vi "MPUAutoReadOn.vi"(8 "ErrorIn(no error)":errorcluster, 10 "SampleRate(1000Hz)":u32=1000, 11 "FPGA VI引用输入":refnum<k20>) -> (0 "ErrorOut":errorcluster, 3 "FPGA VI引用输出":refnum<k20>)   [LabVIEW 2015]
uses:
  <vilib>/Utility/error.llb/Error Cluster From Error Code.vi
  <vilib>/rvi/errors/niLvFpgaAdjustHostInterfaceError.vi
  <vilib>/rvi/interface/nirviReadWriteControl/nirviReadWriteControl.xnode
  NiFpgaLv.dll
  <vilib>/rvi/interface/Simulation/niFpgaSimulationCallBeginRW.vi
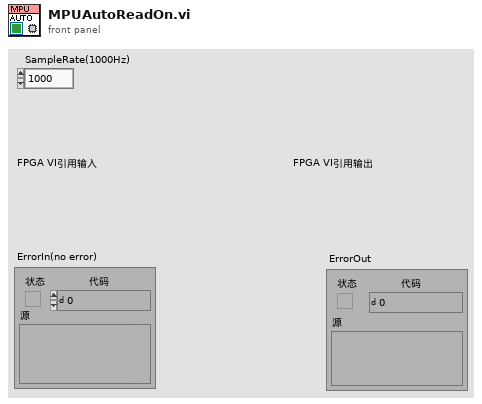
[diagram p1: front panel]
types:
  T1 = enum8{"IDLE", "SetIDLE", "Config", "Arm", "Read", "Write", "AutoRead"}
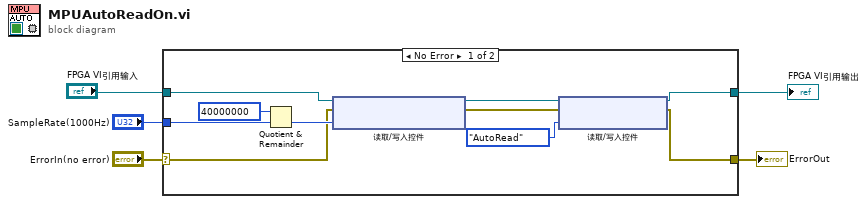
[diagram p0: block diagram]
diagram:
  n1 = case shown="No Error" "ErrorIn(no error)" {
    selector: "ErrorIn(no error)" -> [w8 w16]
    tunnel: "FPGA VI引用输入" -> [w12 w17]
    tunnel: "SampleRate(1000Hz)" -> [w10 _]
    tunnel: [w7 w17] -> w1
    tunnel: [w6 w16] -> w3
    frame No Error {
      n2 = Quotient & Remainder(x=u32 40000000, y=w10) -> (floor(x/y)=w9:u32)  [unwired: 1 out]
      n3 = xnode "读取/写入控件"("FPGA VI Reference In"=w12, "error in"=w8, "SampleRate_Divider"=w9) -> ("FPGA VI Reference Out"=w14:refnum<k20>, "error out"=w13:errorcluster)
      n4 = xnode "读取/写入控件"("FPGA VI Reference In"=w14, "error in"=w13, "ProtocolControl"=T1."AutoRead") -> ("FPGA VI Reference Out"=w7:refnum<k20>, "error out"=w6:errorcluster)
    }
    frame Error {
    }
  }
  "ErrorOut" <- w3
  "FPGA VI引用输出" <- w1
